vi "MassFlowController.vi"() -> ()   [LabVIEW 2017]
uses:
  <vilib>/express/express shared/transition.llb/Dynamic To Waveform Array.vi
  <vilib>/express/express arith-compare/Formula/Block/exnFormulaBlock how many pts in the wave.vi
  <vilib>/express/express shared/ex_Modify Signal Name.vi
  <vilib>/express/express shared/transition.llb/Waveform Array To Dynamic.vi
  <vilib>/express/express arith-compare/Formula/XNode/ExpressFormulaBlockNode.xnode
  <vilib>/addons/control/pid/pid.llb/PID (DBL).vi
  <vilib>/addons/control/pid/NI_PID_pid.lvlib
  <vilib>/addons/control/pid/NI_PID_autopid.lvlib
panel:
  out "Temperature ('C)":dbl
  out "Temperature ('C)":dynamicdata(graph)
  out "Elapsed Time (s)":dbl
  out "Entrance Pressure (kPa)":dbl
  out "Channel Pressure (kPa)":dbl
  in  "PID gains":T1={"proportional gain (Kc)"=1.0, "integral time (Ti, min)"=0.01, "derivative time (Td, min)"=0.0} {"derivative time (Td, min)" format="%.3f"; "integral time (Ti, min)" format="%.3f"; "proportional gain (Kc)" format="%.3f"}
  in  "autotune? (F)":bool
  out "Aim Flow (SLPM)":dbl format="%.2f"
  out "Normal Velocity (m/s)":dbl
  out "Flow (g/s)":dbl
  out "Flow (SLPM)":dbl
  out "?":bool
  out "?":bool
  in  "Flow Controller\n\n\n\n\n\n\n\n\n\n\nPressure Controller":bool
  in  "Pressure (kPa)":dbl(slide) scale=0.0..34.0
  out "Output Signal to Valve (v)":dbl(knob) scale=0.0..5.0
  out "Pressure (kPa)":dynamicdata(graph)
  out "Flow (SLPM)":dynamicdata(graph)
  in  "?":bool
  in  "Flow SetPoint (SLPM)":dbl(slide) scale=0.0..200.0
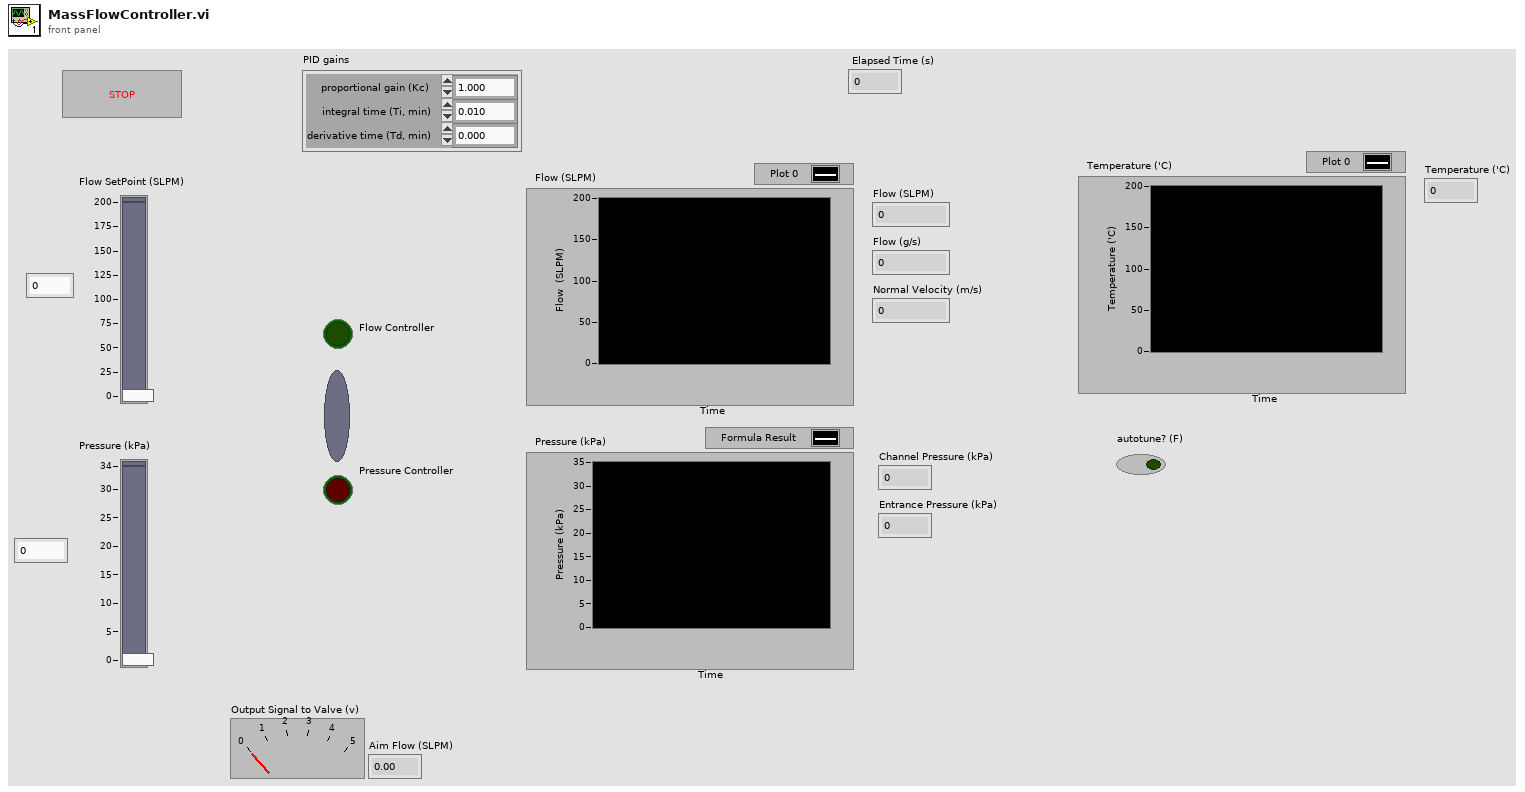
[diagram p1: front panel]
types:
  T1 = cluster{"proportional gain (Kc)":dbl, "integral time (Ti, min)":dbl, "derivative time (Td, min)":dbl}
  T2 = cluster{"controller type":u16, "relay cycles":i32, "relay amplitude":dbl, "control specification":u16, "PV noise level":dbl}
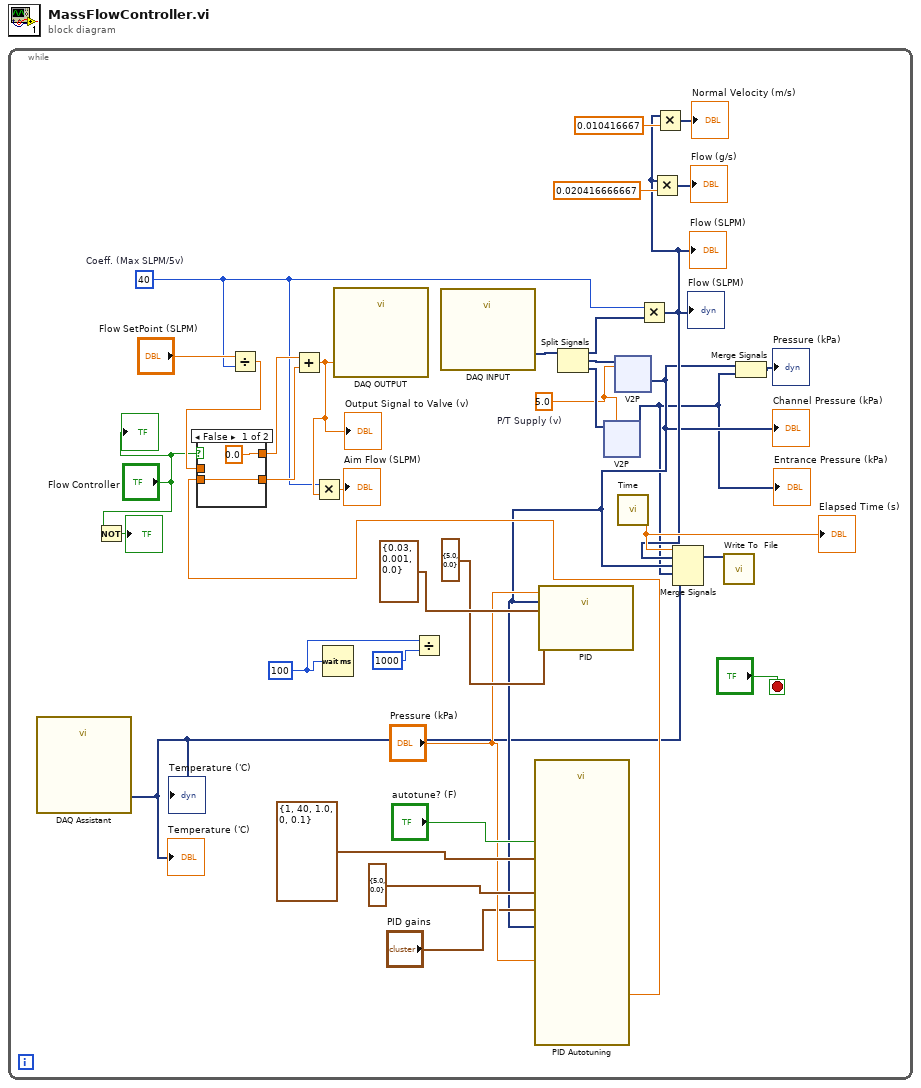
[diagram p0: block diagram]
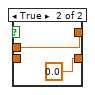
[diagram p2: hidden frame]
diagram:
  n1 = while {
    stop <- "?" stop-if-true
    w13 = u32 100 ("milliseconds to wait")
    w4 = 5.0  # P/T Supply (v)
    w16 = 40  # Coeff. (Max SLPM/5v)
    n2 = call "DAQ Assistant"() -> ("data"=w1:dynamicdata)  [unwired: 17 in, 2 out]
    "Temperature ('C)" <- w1
    "Temperature ('C)" <- w1
    n3 = Not(x="Flow Controller\n\n\n\n\n\n\n\n\n\n\nPressure Controller") -> (.not. x?=→"?":bool)
    n4 = Divide(x="Flow SetPoint (SLPM)", y=w16) -> (x/y=w30:dbl)
    n5 = Wait (ms)(milliseconds to wait=w13) -> ()  [unwired: 1 out]
    n6 = Divide(x=w13, y=u32 1000) -> ()  [unwired: 1 out]
    n7 = call "DAQ INPUT"() -> ("data"=w24:dynamicdata)  [unwired: 17 in, 2 out]
    n8 = Split Signals(w24) -> (w34:dynamicdata, w33:dynamicdata, w5:dynamicdata)  [unwired: 3 in]
    n9 = xnode "V2P"("X1"=w5, "X2"=w4) -> ("Result"=w2:dynamicdata)  [unwired: 1 in, 1 out]
    "Entrance Pressure (kPa)" <- w2
    n10 = xnode "V2P"("X1"=w33, "X2"=w4) -> ("Result"=w3:dynamicdata)  [unwired: 1 in, 1 out]
    "Channel Pressure (kPa)" <- w3
    n11 = call <vilib>:"PID Autotuning.vi"("autotune? (F)"="autotune? (F)", "autotuning parameters"=T2 {"controller type"=1, "relay cycles"=40, "relay amplitude"=1.0, "control specification"=0, "PV noise level"=0.1}, "output range"=cluster{"output high":dbl, "output low":dbl} {"output high"=5.0, "output low"=0.0}, "PID gains"="PID gains", "process variable"=w3, "setpoint"="Pressure (kPa)") -> ("output"=w8:dbl)  [unwired: 2 in, 3 out]
    n12 = case shown="False" "Flow Controller\n\n\n\n\n\n\n\n\n\n\nPressure Controller" {
      tunnel: [0.0 w179] -> w29
      tunnel: w8 -> [w177 _]
      tunnel: [w177 0.0 ("output")] -> w28
      tunnel: w30 -> [_ w179]
      frame False {
      }
      frame True {
      }
    }
    n13 = Add(x=w29, y=w28) -> (x+y=w17:dbl)
    "Output Signal to Valve (v)" <- w17
    n14 = Multiply(x=w16, y=w17) -> (x*y=→"Aim Flow (SLPM)":dbl)
    n15 = call "DAQ OUTPUT"("data"=w17) -> ()  [unwired: 17 in, 2 out]
    n16 = call-poly <vilib>:"PID.vi"("output range"=cluster{"output high":dbl, "output low":dbl} {"output high"=5.0, "output low"=0.0}, "PID gains"=T1 {"proportional gain (Kc)"=0.03, "integral time (Ti, min)"=0.001, "derivative time (Td, min)"=0.0}, "process variable"=w3, "setpoint"="Pressure (kPa)") -> ()  [unwired: 6 in, 2 out]
    n17 = call "Time"() -> ("Elapsed Time (s)"=w23:dbl)  [unwired: 12 in, 7 out]
    "Elapsed Time (s)" <- w23
    n18 = Multiply(x=w16, y=w34) -> (x*y=w15:dynamicdata)
    "Flow (SLPM)" <- w15
    "Flow (SLPM)" <- w15
    n19 = Multiply(x=w15, y=0.020416666667) -> (x*y=→"Flow (g/s)":dynamicdata)
    n20 = Multiply(x=w15, y=0.010416667) -> (x*y=→"Normal Velocity (m/s)":dynamicdata)
    n21 = Merge Signals(w23, w15, w3, w2, w1) -> (w25:dynamicdata)
    n22 = call "Write To  File"("Signals"=w25) -> ()  [unwired: 16 in, 3 out]
    n23 = Merge Signals(w3, w2) -> (→"Pressure (kPa)":dynamicdata)
    "?" <- "Flow Controller\n\n\n\n\n\n\n\n\n\n\nPressure Controller"
  }
